vi "getProtocolName.vi"(11 "CONNECT in":refnum<class "CONNECT.lvclass">) -> (2 "ProtocolName":u8[](array[numeric]) format="%08b", 3 "CONNECT out":refnum<class "CONNECT.lvclass">)   [LabVIEW 2013, in "MQTT_Control_Packets.lvlib" / "CONNECT.lvclass"]
uses:
  CONNECT.lvclass
  ControlPacket/ControlPacket.lvclass
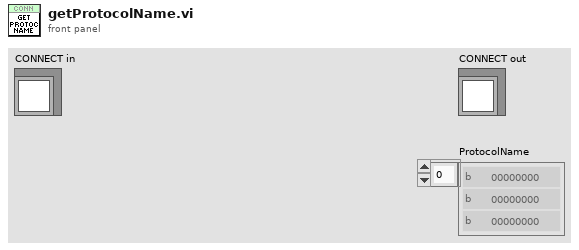
[diagram p1: front panel]
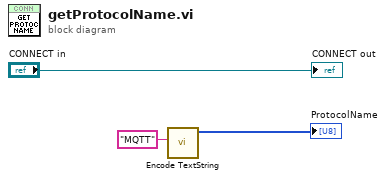
[diagram p0: block diagram]
diagram:
  n1 = call "Encode TextString.vi"("Text String"="MQTT") -> ("Length-Prefixed Field"=→"ProtocolName":u8[])  [unwired: 10 in]
  "CONNECT out" <- "CONNECT in"
